vi "SortMessages.vi"() -> ()   [LabVIEW 2020, in "CTI-Peripheral.lvlib"]
uses:
  CTI-Peripheral.lvlib
  Controls/ASCII.ctl
  Controls/ICONS.ctl
  <vilib>/Utility/error.llb/Trim Whitespace One-Sided.vi
panel:
  out "BytesOut 2":u8[](array[numeric]) format="%.0x"
  in  "stop":bool
  out "Shifting ASCII":bool[][](array[boolean])
  out "8x8Text":bool[][](array[boolean])
  in  "Text":string
  out "element":cluster{"BytesOut":u8[]} {"BytesOut" format="%.0x"}
  out "BytesOut":u8[](array[numeric]) format="%.0x"
  in  "ASCII In":bool[][](array[boolean])
  out "ASCII":bool[][](array[boolean])
  out "Boolean array":bool[][](array[boolean])
  in  "Icons":T1
  in  "ASCII":T2
  out "Array":cluster{"BytesOut":u8[]}[](array[cluster])=[{"BytesOut"=[0, 0, 0, 0, 0, 0, 0, 0]}, {"BytesOut"=[24, 0, 24, 24, 60, 60, 24, 0]}, {"BytesOut"=[0, 0, 0, 0, 40, 108, 108, 0]}, {"BytesOut"=[108, 108, 254, 108, 254, 108, 108, 0]}, {"BytesOut"=[16, 60, 64, 56, 4, 120, 16, 0]}, {"BytesOut"=[96, 102, 12, 24, 48, 102, 6, 0]}, {"BytesOut"=[252, 102, 166, 20, 60, 102, 60, 0]}, {"BytesOut"=[0, 0, 0, 12, 24, 24, 24, 0]}, {"BytesOut"=[96, 48, 24, 24, 24, 48, 96, 0]}, {"BytesOut"=[6, 12, 24, 24, 24, 12, 6, 0]}, {"BytesOut"=[0, 108, 56, 254, 56, 108, 0, 0]}, {"BytesOut"=[0, 16, 16, 124, 16, 16, 0, 0]}, {"BytesOut"=[6, 12, 12, 12, 0, 0, 0, 0]}, {"BytesOut"=[0, 0, 0, 60, 0, 0, 0, 0]}, {"BytesOut"=[6, 6, 0, 0, 0, 0, 0, 0]}, {"BytesOut"=[0, 6, 12, 24, 48, 96, 0, 0]}, {"BytesOut"=[28, 34, 34, 34, 34, 34, 34, 28]}, {"BytesOut"=[28, 8, 8, 8, 8, 8, 12, 8]}, {"BytesOut"=[62, 4, 8, 16, 32, 32, 34, 28]}, {"BytesOut"=[28, 34, 32, 32, 24, 32, 34, 28]}, {"BytesOut"=[32, 32, 62, 34, 36, 40, 48, 32]}, {"BytesOut"=[28, 34, 32, 32, 30, 2, 2, 62]}, {"BytesOut"=[28, 34, 34, 34, 30, 2, 34, 28]}, {"BytesOut"=[4, 4, 4, 8, 16, 32, 32, 62]}, {"BytesOut"=[28, 34, 34, 34, 28, 34, 34, 28]}, {"BytesOut"=[28, 34, 32, 60, 34, 34, 34, 28]}, {"BytesOut"=[0, 24, 24, 0, 24, 24, 0, 0]}, {"BytesOut"=[12, 24, 24, 0, 24, 24, 0, 0]}, {"BytesOut"=[96, 48, 24, 12, 24, 48, 96, 0]}, {"BytesOut"=[0, 0, 60, 0, 60, 0, 0, 0]}, {"BytesOut"=[6, 12, 24, 48, 24, 12, 6, 0]}, {"BytesOut"=[24, 0, 24, 56, 96, 102, 60, 0]}, {"BytesOut"=[0, 60, 66, 26, 58, 34, 28, 0]}, {"BytesOut"=[0, 51, 51, 63, 51, 51, 30, 12]}, {"BytesOut"=[0, 63, 102, 102, 62, 102, 102, 63]}, {"BytesOut"=[0, 60, 102, 3, 3, 3, 102, 60]}, {"BytesOut"=[0, 31, 54, 102, 102, 102, 54, 31]}, {"BytesOut"=[0, 127, 70, 22, 30, 22, 70, 127]}, {"BytesOut"=[0, 15, 6, 22, 30, 22, 70, 127]}, {"BytesOut"=[0, 124, 102, 115, 3, 3, 102, 60]}, {"BytesOut"=[0, 51, 51, 51, 63, 51, 51, 51]}, {"BytesOut"=[0, 30, 12, 12, 12, 12, 12, 30]}, {"BytesOut"=[0, 30, 51, 51, 48, 48, 48, 120]}, {"BytesOut"=[0, 103, 102, 54, 30, 54, 102, 103]}, {"BytesOut"=[0, 127, 102, 70, 6, 6, 6, 15]}, {"BytesOut"=[0, 99, 99, 107, 127, 127, 119, 99]}, {"BytesOut"=[0, 99, 99, 115, 123, 111, 103, 99]}, {"BytesOut"=[0, 28, 54, 99, 99, 99, 54, 28]}, {"BytesOut"=[0, 15, 6, 6, 62, 102, 102, 63]}, {"BytesOut"=[0, 56, 30, 59, 51, 51, 51, 30]}, {"BytesOut"=[0, 103, 102, 54, 62, 102, 102, 63]}, {"BytesOut"=[0, 30, 51, 56, 14, 7, 51, 30]}, {"BytesOut"=[0, 30, 12, 12, 12, 12, 45, 63]}, {"BytesOut"=[0, 63, 51, 51, 51, 51, 51, 51]}, {"BytesOut"=[0, 12, 30, 51, 51, 51, 51, 51]}, {"BytesOut"=[0, 99, 119, 127, 107, 99, 99, 99]}, {"BytesOut"=[0, 99, 54, 28, 28, 54, 99, 99]}, {"BytesOut"=[0, 30, 12, 12, 30, 51, 51, 51]}, {"BytesOut"=[0, 127, 102, 76, 24, 49, 99, 127]}, {"BytesOut"=[120, 24, 24, 24, 24, 24, 120, 0]}, {"BytesOut"=[0, 96, 48, 24, 12, 6, 0, 0]}, {"BytesOut"=[30, 24, 24, 24, 24, 24, 30, 0]}, {"BytesOut"=[0, 0, 0, 130, 68, 40, 16, 0]}, {"BytesOut"=[126, 0, 0, 0, 0, 0, 0, 0]}, {"BytesOut"=[0, 0, 0, 0, 96, 48, 48, 0]}, {"BytesOut"=[0, 110, 51, 62, 48, 30, 0, 0]}, {"BytesOut"=[0, 59, 102, 102, 62, 6, 6, 7]}, {"BytesOut"=[0, 30, 51, 3, 51, 30, 0, 0]}, {"BytesOut"=[0, 110, 51, 51, 62, 48, 48, 56]}, {"BytesOut"=[0, 30, 3, 63, 51, 30, 0, 0]}, {"BytesOut"=[0, 15, 6, 6, 15, 6, 54, 28]}, {"BytesOut"=[31, 48, 62, 51, 51, 110, 0, 0]}, {"BytesOut"=[0, 103, 102, 102, 110, 54, 6, 7]}, {"BytesOut"=[0, 30, 12, 12, 12, 14, 0, 12]}, {"BytesOut"=[30, 51, 51, 48, 48, 48, 0, 48]}, {"BytesOut"=[0, 103, 54, 30, 54, 102, 6, 7]}, {"BytesOut"=[0, 30, 12, 12, 12, 12, 12, 14]}, {"BytesOut"=[0, 99, 107, 127, 127, 51, 0, 0]}, {"BytesOut"=[0, 51, 51, 51, 51, 31, 0, 0]}, {"BytesOut"=[0, 30, 51, 51, 51, 30, 0, 0]}, {"BytesOut"=[15, 6, 62, 102, 102, 59, 0, 0]}, {"BytesOut"=[120, 48, 62, 51, 51, 110, 0, 0]}, {"BytesOut"=[0, 15, 6, 102, 110, 59, 0, 0]}, {"BytesOut"=[0, 31, 48, 30, 3, 62, 0, 0]}, {"BytesOut"=[0, 24, 44, 12, 12, 62, 12, 8]}, {"BytesOut"=[0, 110, 51, 51, 51, 51, 0, 0]}, {"BytesOut"=[0, 12, 30, 51, 51, 51, 0, 0]}, {"BytesOut"=[0, 54, 127, 127, 107, 99, 0, 0]}, {"BytesOut"=[0, 99, 54, 28, 54, 99, 0, 0]}, {"BytesOut"=[31, 48, 62, 51, 51, 51, 0, 0]}, {"BytesOut"=[0, 63, 38, 12, 25, 63, 0, 0]}, {"BytesOut"=[112, 24, 24, 12, 24, 24, 112, 0]}, {"BytesOut"=[0, 8, 8, 8, 8, 8, 8, 0]}, {"BytesOut"=[14, 24, 24, 48, 24, 24, 14, 0]}, {"BytesOut"=[0, 0, 0, 54, 92, 0, 0, 0, 0, 0, 0, 0, 0]}] {"BytesOut" format="%.0x"}
  out "unsigned byte array":u8[](array[numeric])
  out "array":string[](array[string])=[" 0x0000000000000000,     // space", "    0x180018183c3c1800,     // !", "    0x00000000286c6c00,     // \"", "    0x6c6cfe6cfe6c6c00,     // #", "    0x103c403804781000,     // $", "    0x60660c1830660600,     // %", "    0xfc66a6143c663c00,     // &", "    0x0000000c18181800,     // '", "    0x6030181818306000,     // (", "    0x060c1818180c0600,     // )", "    0x006c38fe386c0000,     // *", "    0x0010107c10100000,     // +", "    0x060c0c0c00000000,     // ,", "    0x0000003c00000000,     // -", "    0x0606000000000000,     // .", "    0x00060c1830600000,     // /", "    0x1c2222222222221c,     // 0", "    0x1c08080808080c08,     // 1", "    0x3e0408102020221c,     // 2", "    0x1c2220201820221c,     // 3", "    0x20203e2224283020,     // 4", "    0x1c2220201e02023e,     // 5", "    0x1c2222221e02221c,     // 6", "    0x040404081020203e,     // 7", "    0x1c2222221c22221c,     // 8", "    0x1c22203c2222221c,     // 9", "    0x0018180018180000,     // :", "    0x0c18180018180000,     // ;", "    0x6030180c18306000,     // <", "    0x00003c003c000000,     // =", "    0x060c1830180c0600,     // >", "    0x1800183860663c00,     // ?", "    0x003c421a3a221c00,     // @", "    0x0033333f33331e0c,     // A", "    0x003f66663e66663f,     // B", "    0x003c66030303663c,     // C", "    0x001f36666666361f,     // D", "    0x007f46161e16467f,     // E", "    0x000f06161e16467f,     // F", "    0x007c66730303663c,     // G", "    0x003333333f333333,     // H", "    0x001e0c0c0c0c0c1e,     // I", "    0x001e333330303078,     // J", "    0x006766361e366667,     // K", "    0x007f66460606060f,     // L", "    0x0063636b7f7f7763,     // M", "    0x006363737b6f6763,     // N", "    0x001c36636363361c,     // O", "    0x000f06063e66663f,     // P", "    0x00381e3b3333331e,     // Q", "    0x006766363e66663f,     // R", "    0x001e33380e07331e,     // S", "    0x001e0c0c0c0c2d3f,     // T", "    0x003f333333333333,     // U", "    0x000c1e3333333333,     // V", "    0x0063777f6b636363,     // W", "    0x0063361c1c366363,     // X", "    0x001e0c0c1e333333,     // Y", "    0x007f664c1831637f,     // Z", "    0x7818181818187800,     // [", "    0x006030180c060000,     // '\\'", "    0x1e18181818181e00,     // ]", "    0x0000008244281000,     // ^", "    0x7e00000000000000,     // _", "    0x0000000060303000,     // `", "    0x006e333e301e0000,     // a", "    0x003b66663e060607,     // b", "    0x001e3303331e0000,     // c", "    0x006e33333e303038,     // d", "    0x001e033f331e0000,     // e", "    0x000f06060f06361c,     // f", "    0x1f303e33336e0000,     // g", "    0x006766666e360607,     // h", "    0x001e0c0c0c0e000c,     // i", "    0x1e33333030300030,     // j", "    0x0067361e36660607,     // k", "    0x001e0c0c0c0c0c0e,     // l", "    0x00636b7f7f330000,     // m", "    0x00333333331f0000,     // n", "    0x001e3333331e0000,     // o", "    0x0f063e66663b0000,     // p", "    0x78303e33336e0000,     // q", "    0x000f06666e3b0000,     // r", "    0x001f301e033e0000,     // s", "    0x00182c0c0c3e0c08,     // t", "    0x006e333333330000,     // u", "    0x000c1e3333330000,     // v", "    0x00367f7f6b630000,     // w", "    0x0063361c36630000,     // x", "    0x1f303e3333330000,     // y", "    0x003f260c193f0000,     // z", "    0x7018180c18187000,     // {", "    0x0008080808080800,     // |", "    0x0e18183018180e00,     // }", "    0x000000365c000000      // ~"]
  in  "String":string=" 0x0000000000000000,     // space\n    0x180018183c3c1800,     // !\n    0x00000000286c6c00,     // \"\n    0x6c6cfe6cfe6c6c00,     // #\n    0x103c403804781000,     // $\n    0x60660c1830660600,     // %\n    0xfc66a6143c663c00,     // &\n    0x0000000c18181800,     // '\n    0x6030181818306000,     // (\n    0x060c1818180c0600,     // )\n    0x006c38fe386c0000,     // *\n    0x0010107c10100000,     // +\n    0x060c0c0c00000000,     // ,\n    0x0000003c00000000,     // -\n    0x0606000000000000,     // .\n    0x00060c1830600000,     // /\n    0x1c2222222222221c,     // 0\n    0x1c08080808080c08,     // 1\n    0x3e0408102020221c,     // 2\n    0x1c2220201820221c,     // 3\n    0x20203e2224283020,     // 4\n    0x1c2220201e02023e,     // 5\n    0x1c2222221e02221c,     // 6\n    0x040404081020203e,     // 7\n    0x1c2222221c22221c,     // 8\n    0x1c22203c2222221c,     // 9\n    0x0018180018180000,     // :\n    0x0c18180018180000,     // ;\n    0x6030180c18306000,     // <\n    0x00003c003c000000,     // =\n    0x060c1830180c0600,     // >\n    0x1800183860663c00,     // ?\n    0x003c421a3a221c00,     // @\n    0x0033333f33331e0c,     // A\n    0x003f66663e66663f,     // B\n    0x003c66030303663c,     // C\n    0x001f36666666361f,     // D\n    0x007f46161e16467f,     // E\n    0x000f06161e16467f,     // F\n    0x007c66730303663c,     // G\n    0x003333333f333333,     // H\n    0x001e0c0c0c0c0c1e,     // I\n    0x001e333330303078,     // J\n    0x006766361e366667,     // K\n    0x007f66460606060f,     // L\n    0x0063636b7f7f7763,     // M\n    0x006363737b6f6763,     // N\n    0x001c36636363361c,     // O\n    0x000f06063e66663f,     // P\n    0x00381e3b3333331e,     // Q\n    0x006766363e66663f,     // R\n    0x001e33380e07331e,     // S\n    0x001e0c0c0c0c2d3f,     // T\n    0x003f333333333333,     // U\n    0x000c1e3333333333,     // V\n    0x0063777f6b636363,     // W\n    0x0063361c1c366363,     // X\n    0x001e0c0c1e333333,     // Y\n    0x007f664c1831637f,     // Z\n    0x7818181818187800,     // [\n    0x006030180c060000,     // '\\'\n    0x1e18181818181e00,     // ]\n    0x0000008244281000,     // ^\n    0x7e00000000000000,     // _\n    0x0000000060303000,     // `\n    0x006e333e301e0000,     // a\n    0x003b66663e060607,     // b\n    0x001e3303331e0000,     // c\n    0x006e33333e303038,     // d\n    0x001e033f331e0000,     // e\n    0x000f06060f06361c,     // f\n    0x1f303e33336e0000,     // g\n    0x006766666e360607,     // h\n    0x001e0c0c0c0e000c,     // i\n    0x1e33333030300030,     // j\n    0x0067361e36660607,     // k\n    0x001e0c0c0c0c0c0e,     // l\n    0x00636b7f7f330000,     // m\n    0x00333333331f0000,     // n\n    0x001e3333331e0000,     // o\n    0x0f063e66663b0000,     // p\n    0x78303e33336e0000,     // q\n    0x000f06666e3b0000,     // r\n    0x001f301e033e0000,     // s\n    0x00182c0c0c3e0c08,     // t\n    0x006e333333330000,     // u\n    0x000c1e3333330000,     // v\n    0x00367f7f6b630000,     // w\n    0x0063361c36630000,     // x\n    0x1f303e3333330000,     // y\n    0x003f260c193f0000,     // z\n    0x7018180c18187000,     // {\n    0x0008080808080800,     // |\n    0x0e18183018180e00,     // }\n    0x000000365c000000      // ~"
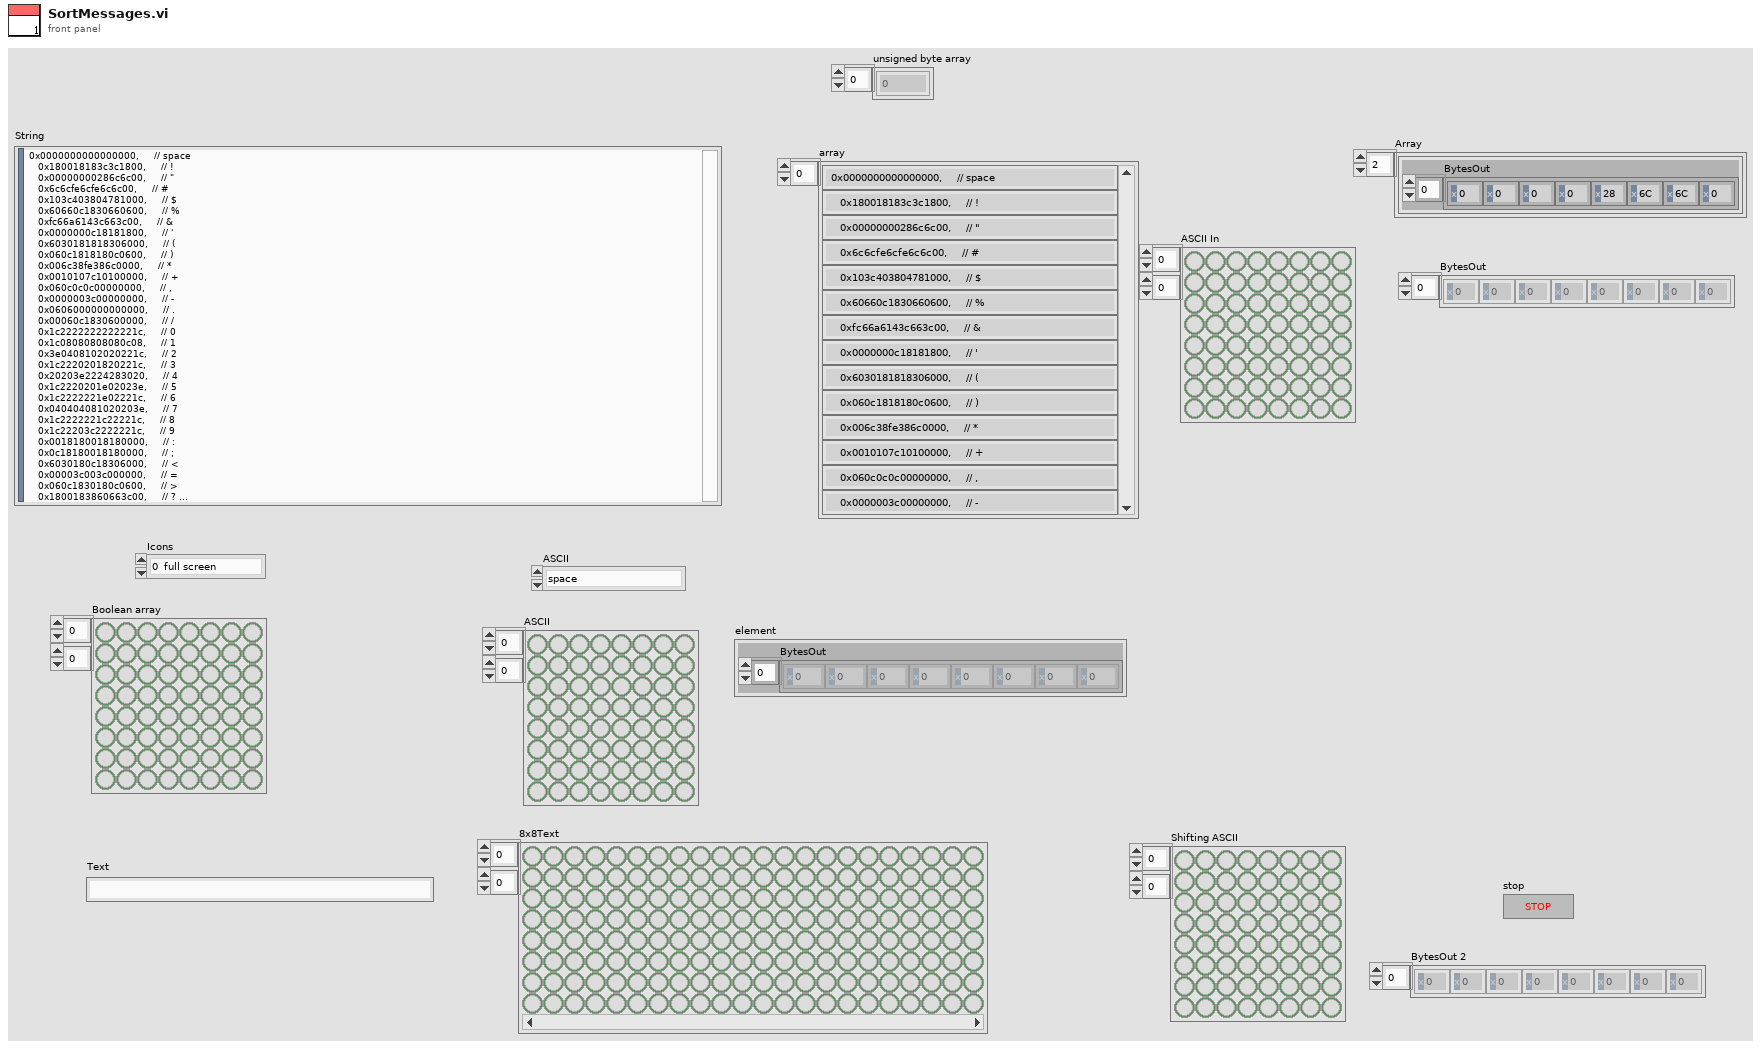
[diagram p1: front panel]
types:
  T1 = typedef "ICONS.ctl" = enum16{"0  full screen", "1  arrow_up", "2  arrow_down", "3  arrow_right", "4  arrow_left", "5  triangle_up", "6  triangle_down", "7  triangle_right", "8  triangel_left", "9  smile_face_1", "10 smile_face_2", "11 hearts", "12 diamonds", "13 clubs", "14 spades", "15 circle1", "16 circle2", "17 circle3", "18 circle4", "19 man", "20 woman", "21 musical_note_1", "22 musical_note_2", "23 snow", "24 up_down", "25 double_!", "26 left_right", "27 house"}
  T2 = typedef "CTI-Peripheral.lvlib/ASCII.ctl" = enum16{"space", "!", "\"", "#", "$", "%", "&", "'", "(", ")", "*", "+", ",", "- ", ".", "/", "0", "1", "2", "3", "4", "5", "6", "7", "8", "9", ":", ";", "<", "=", ">", "?", "@", "A", "B", "C", "D", "E", "F", "G", "H", "I", "J", "K", "L", "M", "N", "O", "P", "Q", "R", "S", "T", "U", "V", "W", "X", "Y", "Z", "[", "'\\'", "]", "^", "_", "`", "a", "b", "c", "d", "e", "f", "g", "h", "i", "j", "k", "l", "m", "n", "o", "p", "q", "r", "s", "t", "u", "v", "w", "x", "y", "z", "{", "|", "}", ""}
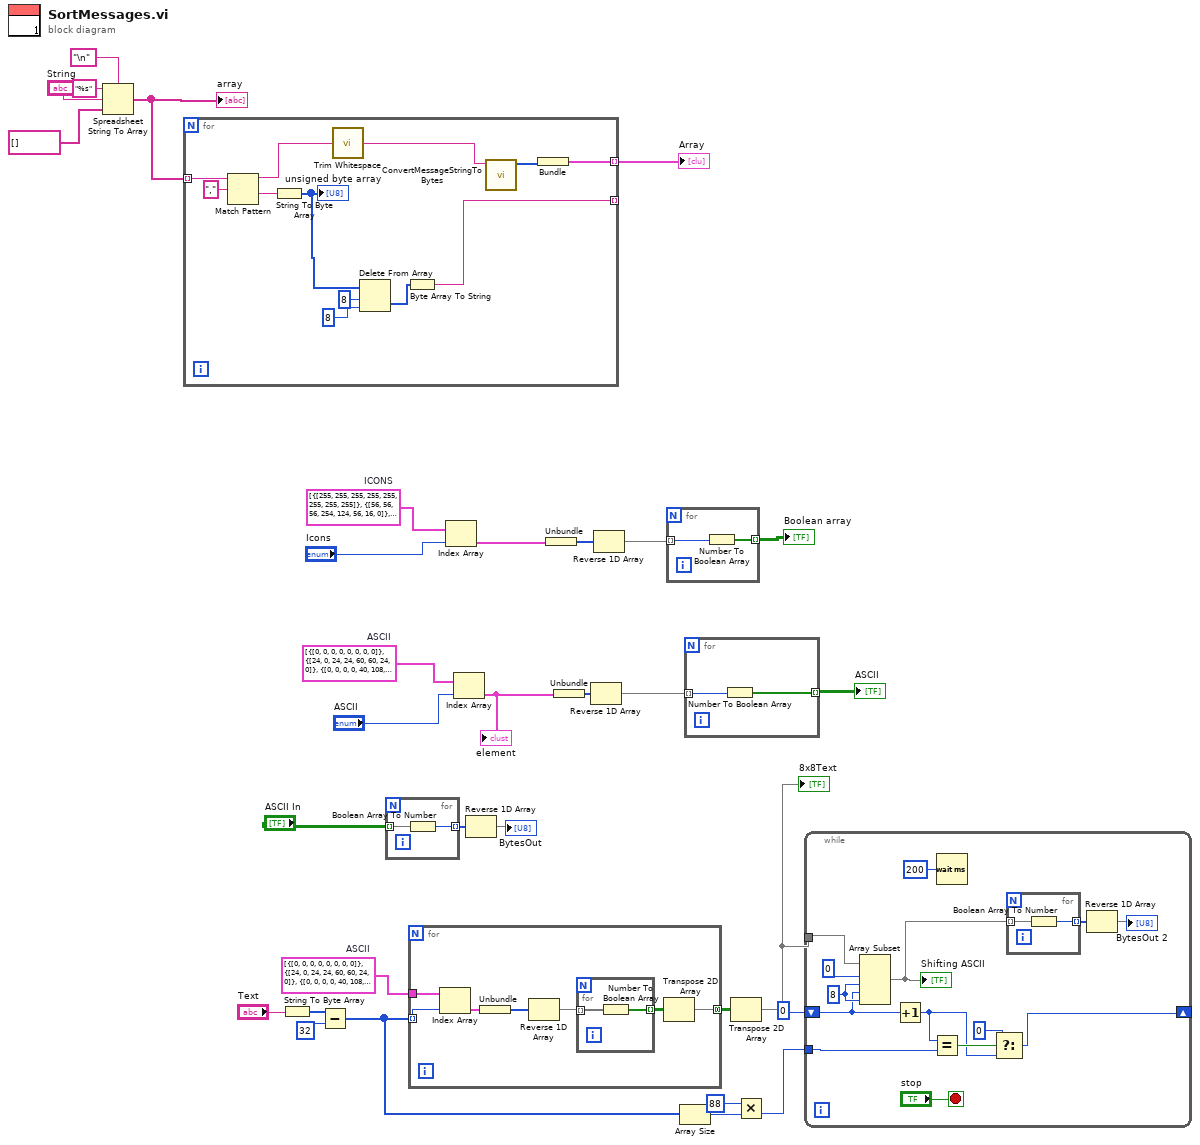
[diagram p0: block diagram]
diagram:
  w8 = cluster{"BytesOut":u8[]}[] [{"BytesOut"=[0, 0, 0, 0, 0, 0, 0, 0]}, {"BytesOut"=[24, 0, 24, 24, 60, 60, 24, 0]}, {"BytesOut"=[0, 0, 0, 0, 40, 108, 108, 0]}, {"BytesOut"=[108, 108, 254, 108, 254, 108, 108, 0]}, {"BytesOut"=[16, 60, 64, 56, 4, 120, 16, 0]}, {"BytesOut"=[96, 102, 12, 24, 48, 102, 6, 0]}, {"BytesOut"=[252, 102, 166, 20, 60, 102, 60, 0]}, {"BytesOut"=[0, 0, 0, 12, 24, 24, 24, 0]}, {"BytesOut"=[96, 48, 24, 24, 24, 48, 96, 0]}, {"BytesOut"=[6, 12, 24, 24, 24, 12, 6, 0]}, {"BytesOut"=[0, 108, 56, 254, 56, 108, 0, 0]}, {"BytesOut"=[0, 16, 16, 124, 16, 16, 0, 0]}, {"BytesOut"=[6, 12, 12, 12, 0, 0, 0, 0]}, {"BytesOut"=[0, 0, 0, 60, 0, 0, 0, 0]}, {"BytesOut"=[6, 6, 0, 0, 0, 0, 0, 0]}, {"BytesOut"=[0, 6, 12, 24, 48, 96, 0, 0]}, {"BytesOut"=[28, 34, 34, 34, 34, 34, 34, 28]}, {"BytesOut"=[28, 8, 8, 8, 8, 8, 12, 8]}, {"BytesOut"=[62, 4, 8, 16, 32, 32, 34, 28]}, {"BytesOut"=[28, 34, 32, 32, 24, 32, 34, 28]}, {"BytesOut"=[32, 32, 62, 34, 36, 40, 48, 32]}, {"BytesOut"=[28, 34, 32, 32, 30, 2, 2, 62]}, {"BytesOut"=[28, 34, 34, 34, 30, 2, 34, 28]}, {"BytesOut"=[4, 4, 4, 8, 16, 32, 32, 62]}, {"BytesOut"=[28, 34, 34, 34, 28, 34, 34, 28]}, {"BytesOut"=[28, 34, 32, 60, 34, 34, 34, 28]}, {"BytesOut"=[0, 24, 24, 0, 24, 24, 0, 0]}, {"BytesOut"=[12, 24, 24, 0, 24, 24, 0, 0]}, {"BytesOut"=[96, 48, 24, 12, 24, 48, 96, 0]}, {"BytesOut"=[0, 0, 60, 0, 60, 0, 0, 0]}, {"BytesOut"=[6, 12, 24, 48, 24, 12, 6, 0]}, {"BytesOut"=[24, 0, 24, 56, 96, 102, 60, 0]}, {"BytesOut"=[0, 60, 66, 26, 58, 34, 28, 0]}, {"BytesOut"=[0, 51, 51, 63, 51, 51, 30, 12]}, {"BytesOut"=[0, 63, 102, 102, 62, 102, 102, 63]}, {"BytesOut"=[0, 60, 102, 3, 3, 3, 102, 60]}, {"BytesOut"=[0, 31, 54, 102, 102, 102, 54, 31]}, {"BytesOut"=[0, 127, 70, 22, 30, 22, 70, 127]}, {"BytesOut"=[0, 15, 6, 22, 30, 22, 70, 127]}, {"BytesOut"=[0, 124, 102, 115, 3, 3, 102, 60]}, {"BytesOut"=[0, 51, 51, 51, 63, 51, 51, 51]}, {"BytesOut"=[0, 30, 12, 12, 12, 12, 12, 30]}, {"BytesOut"=[0, 30, 51, 51, 48, 48, 48, 120]}, {"BytesOut"=[0, 103, 102, 54, 30, 54, 102, 103]}, {"BytesOut"=[0, 127, 102, 70, 6, 6, 6, 15]}, {"BytesOut"=[0, 99, 99, 107, 127, 127, 119, 99]}, {"BytesOut"=[0, 99, 99, 115, 123, 111, 103, 99]}, {"BytesOut"=[0, 28, 54, 99, 99, 99, 54, 28]}, {"BytesOut"=[0, 15, 6, 6, 62, 102, 102, 63]}, {"BytesOut"=[0, 56, 30, 59, 51, 51, 51, 30]}, {"BytesOut"=[0, 103, 102, 54, 62, 102, 102, 63]}, {"BytesOut"=[0, 30, 51, 56, 14, 7, 51, 30]}, {"BytesOut"=[0, 30, 12, 12, 12, 12, 45, 63]}, {"BytesOut"=[0, 63, 51, 51, 51, 51, 51, 51]}, {"BytesOut"=[0, 12, 30, 51, 51, 51, 51, 51]}, {"BytesOut"=[0, 99, 119, 127, 107, 99, 99, 99]}, {"BytesOut"=[0, 99, 54, 28, 28, 54, 99, 99]}, {"BytesOut"=[0, 30, 12, 12, 30, 51, 51, 51]}, {"BytesOut"=[0, 127, 102, 76, 24, 49, 99, 127]}, {"BytesOut"=[120, 24, 24, 24, 24, 24, 120, 0]}, {"BytesOut"=[0, 96, 48, 24, 12, 6, 0, 0]}, {"BytesOut"=[30, 24, 24, 24, 24, 24, 30, 0]}, {"BytesOut"=[0, 0, 0, 130, 68, 40, 16, 0]}, {"BytesOut"=[126, 0, 0, 0, 0, 0, 0, 0]}, {"BytesOut"=[0, 0, 0, 0, 96, 48, 48, 0]}, {"BytesOut"=[0, 110, 51, 62, 48, 30, 0, 0]}, {"BytesOut"=[0, 59, 102, 102, 62, 6, 6, 7]}, {"BytesOut"=[0, 30, 51, 3, 51, 30, 0, 0]}, {"BytesOut"=[0, 110, 51, 51, 62, 48, 48, 56]}, {"BytesOut"=[0, 30, 3, 63, 51, 30, 0, 0]}, {"BytesOut"=[0, 15, 6, 6, 15, 6, 54, 28]}, {"BytesOut"=[31, 48, 62, 51, 51, 110, 0, 0]}, {"BytesOut"=[0, 103, 102, 102, 110, 54, 6, 7]}, {"BytesOut"=[0, 30, 12, 12, 12, 14, 0, 12]}, {"BytesOut"=[30, 51, 51, 48, 48, 48, 0, 48]}, {"BytesOut"=[0, 103, 54, 30, 54, 102, 6, 7]}, {"BytesOut"=[0, 30, 12, 12, 12, 12, 12, 14]}, {"BytesOut"=[0, 99, 107, 127, 127, 51, 0, 0]}, {"BytesOut"=[0, 51, 51, 51, 51, 31, 0, 0]}, {"BytesOut"=[0, 30, 51, 51, 51, 30, 0, 0]}, {"BytesOut"=[15, 6, 62, 102, 102, 59, 0, 0]}, {"BytesOut"=[120, 48, 62, 51, 51, 110, 0, 0]}, {"BytesOut"=[0, 15, 6, 102, 110, 59, 0, 0]}, {"BytesOut"=[0, 31, 48, 30, 3, 62, 0, 0]}, {"BytesOut"=[0, 24, 44, 12, 12, 62, 12, 8]}, {"BytesOut"=[0, 110, 51, 51, 51, 51, 0, 0]}, {"BytesOut"=[0, 12, 30, 51, 51, 51, 0, 0]}, {"BytesOut"=[0, 54, 127, 127, 107, 99, 0, 0]}, {"BytesOut"=[0, 99, 54, 28, 54, 99, 0, 0]}, {"BytesOut"=[31, 48, 62, 51, 51, 51, 0, 0]}, {"BytesOut"=[0, 63, 38, 12, 25, 63, 0, 0]}, {"BytesOut"=[112, 24, 24, 12, 24, 24, 112, 0]}, {"BytesOut"=[0, 8, 8, 8, 8, 8, 8, 0]}, {"BytesOut"=[14, 24, 24, 48, 24, 24, 14, 0]}, {"BytesOut"=[0, 0, 0, 54, 92, 0, 0, 0, 0, 0, 0, 0, 0]}]  # ASCII
  w26 = cluster{"BytesOut":u8[]}[] [{"BytesOut"=[255, 255, 255, 255, 255, 255, 255, 255]}, {"BytesOut"=[56, 56, 56, 254, 124, 56, 16, 0]}, {"BytesOut"=[16, 56, 124, 254, 56, 56, 56, 0]}, {"BytesOut"=[16, 48, 126, 254, 126, 48, 16, 0]}, {"BytesOut"=[16, 24, 252, 254, 252, 24, 16, 0]}, {"BytesOut"=[254, 254, 124, 124, 56, 56, 16, 0]}, {"BytesOut"=[16, 56, 56, 124, 124, 254, 254, 0]}, {"BytesOut"=[6, 30, 126, 254, 126, 30, 6, 0]}, {"BytesOut"=[192, 240, 252, 254, 252, 240, 192, 0]}, {"BytesOut"=[124, 146, 170, 130, 170, 130, 124, 0]}, {"BytesOut"=[0, 60, 66, 0, 0, 102, 0, 0]}, {"BytesOut"=[16, 56, 124, 254, 254, 238, 68, 0]}, {"BytesOut"=[16, 56, 124, 254, 124, 56, 16, 0]}, {"BytesOut"=[56, 16, 84, 254, 84, 56, 16, 0]}, {"BytesOut"=[56, 16, 124, 254, 124, 56, 16, 0]}, {"BytesOut"=[0, 56, 124, 124, 124, 56, 0, 0]}, {"BytesOut"=[255, 199, 131, 131, 131, 199, 255, 255]}, {"BytesOut"=[0, 56, 68, 68, 68, 56, 0, 0]}, {"BytesOut"=[255, 199, 187, 187, 187, 199, 255, 255]}, {"BytesOut"=[12, 18, 18, 156, 160, 192, 240, 0]}, {"BytesOut"=[56, 68, 68, 56, 16, 124, 16, 0]}, {"BytesOut"=[6, 14, 12, 8, 8, 40, 24, 0]}, {"BytesOut"=[6, 110, 236, 200, 136, 152, 240, 0]}, {"BytesOut"=[16, 84, 56, 238, 56, 84, 16, 0]}, {"BytesOut"=[16, 56, 84, 16, 84, 56, 16, 0]}, {"BytesOut"=[102, 102, 0, 102, 102, 102, 102, 0]}, {"BytesOut"=[0, 40, 68, 254, 68, 40, 0, 0]}, {"BytesOut"=[254, 130, 130, 198, 108, 56, 16, 0]}, {"BytesOut"=[0, 36, 0, 231, 165, 189, 231, 0, 0, 0, 0, 0, 2, 8, 0, 10, 0]}]  # ICONS
  w19 = cluster{"BytesOut":u8[]}[] [{"BytesOut"=[0, 0, 0, 0, 0, 0, 0, 0]}, {"BytesOut"=[24, 0, 24, 24, 60, 60, 24, 0]}, {"BytesOut"=[0, 0, 0, 0, 40, 108, 108, 0]}, {"BytesOut"=[108, 108, 254, 108, 254, 108, 108, 0]}, {"BytesOut"=[16, 60, 64, 56, 4, 120, 16, 0]}, {"BytesOut"=[96, 102, 12, 24, 48, 102, 6, 0]}, {"BytesOut"=[252, 102, 166, 20, 60, 102, 60, 0]}, {"BytesOut"=[0, 0, 0, 12, 24, 24, 24, 0]}, {"BytesOut"=[96, 48, 24, 24, 24, 48, 96, 0]}, {"BytesOut"=[6, 12, 24, 24, 24, 12, 6, 0]}, {"BytesOut"=[0, 108, 56, 254, 56, 108, 0, 0]}, {"BytesOut"=[0, 16, 16, 124, 16, 16, 0, 0]}, {"BytesOut"=[6, 12, 12, 12, 0, 0, 0, 0]}, {"BytesOut"=[0, 0, 0, 60, 0, 0, 0, 0]}, {"BytesOut"=[6, 6, 0, 0, 0, 0, 0, 0]}, {"BytesOut"=[0, 6, 12, 24, 48, 96, 0, 0]}, {"BytesOut"=[28, 34, 34, 34, 34, 34, 34, 28]}, {"BytesOut"=[28, 8, 8, 8, 8, 8, 12, 8]}, {"BytesOut"=[62, 4, 8, 16, 32, 32, 34, 28]}, {"BytesOut"=[28, 34, 32, 32, 24, 32, 34, 28]}, {"BytesOut"=[32, 32, 62, 34, 36, 40, 48, 32]}, {"BytesOut"=[28, 34, 32, 32, 30, 2, 2, 62]}, {"BytesOut"=[28, 34, 34, 34, 30, 2, 34, 28]}, {"BytesOut"=[4, 4, 4, 8, 16, 32, 32, 62]}, {"BytesOut"=[28, 34, 34, 34, 28, 34, 34, 28]}, {"BytesOut"=[28, 34, 32, 60, 34, 34, 34, 28]}, {"BytesOut"=[0, 24, 24, 0, 24, 24, 0, 0]}, {"BytesOut"=[12, 24, 24, 0, 24, 24, 0, 0]}, {"BytesOut"=[96, 48, 24, 12, 24, 48, 96, 0]}, {"BytesOut"=[0, 0, 60, 0, 60, 0, 0, 0]}, {"BytesOut"=[6, 12, 24, 48, 24, 12, 6, 0]}, {"BytesOut"=[24, 0, 24, 56, 96, 102, 60, 0]}, {"BytesOut"=[0, 60, 66, 26, 58, 34, 28, 0]}, {"BytesOut"=[0, 51, 51, 63, 51, 51, 30, 12]}, {"BytesOut"=[0, 63, 102, 102, 62, 102, 102, 63]}, {"BytesOut"=[0, 60, 102, 3, 3, 3, 102, 60]}, {"BytesOut"=[0, 31, 54, 102, 102, 102, 54, 31]}, {"BytesOut"=[0, 127, 70, 22, 30, 22, 70, 127]}, {"BytesOut"=[0, 15, 6, 22, 30, 22, 70, 127]}, {"BytesOut"=[0, 124, 102, 115, 3, 3, 102, 60]}, {"BytesOut"=[0, 51, 51, 51, 63, 51, 51, 51]}, {"BytesOut"=[0, 30, 12, 12, 12, 12, 12, 30]}, {"BytesOut"=[0, 30, 51, 51, 48, 48, 48, 120]}, {"BytesOut"=[0, 103, 102, 54, 30, 54, 102, 103]}, {"BytesOut"=[0, 127, 102, 70, 6, 6, 6, 15]}, {"BytesOut"=[0, 99, 99, 107, 127, 127, 119, 99]}, {"BytesOut"=[0, 99, 99, 115, 123, 111, 103, 99]}, {"BytesOut"=[0, 28, 54, 99, 99, 99, 54, 28]}, {"BytesOut"=[0, 15, 6, 6, 62, 102, 102, 63]}, {"BytesOut"=[0, 56, 30, 59, 51, 51, 51, 30]}, {"BytesOut"=[0, 103, 102, 54, 62, 102, 102, 63]}, {"BytesOut"=[0, 30, 51, 56, 14, 7, 51, 30]}, {"BytesOut"=[0, 30, 12, 12, 12, 12, 45, 63]}, {"BytesOut"=[0, 63, 51, 51, 51, 51, 51, 51]}, {"BytesOut"=[0, 12, 30, 51, 51, 51, 51, 51]}, {"BytesOut"=[0, 99, 119, 127, 107, 99, 99, 99]}, {"BytesOut"=[0, 99, 54, 28, 28, 54, 99, 99]}, {"BytesOut"=[0, 30, 12, 12, 30, 51, 51, 51]}, {"BytesOut"=[0, 127, 102, 76, 24, 49, 99, 127]}, {"BytesOut"=[120, 24, 24, 24, 24, 24, 120, 0]}, {"BytesOut"=[0, 96, 48, 24, 12, 6, 0, 0]}, {"BytesOut"=[30, 24, 24, 24, 24, 24, 30, 0]}, {"BytesOut"=[0, 0, 0, 130, 68, 40, 16, 0]}, {"BytesOut"=[126, 0, 0, 0, 0, 0, 0, 0]}, {"BytesOut"=[0, 0, 0, 0, 96, 48, 48, 0]}, {"BytesOut"=[0, 110, 51, 62, 48, 30, 0, 0]}, {"BytesOut"=[0, 59, 102, 102, 62, 6, 6, 7]}, {"BytesOut"=[0, 30, 51, 3, 51, 30, 0, 0]}, {"BytesOut"=[0, 110, 51, 51, 62, 48, 48, 56]}, {"BytesOut"=[0, 30, 3, 63, 51, 30, 0, 0]}, {"BytesOut"=[0, 15, 6, 6, 15, 6, 54, 28]}, {"BytesOut"=[31, 48, 62, 51, 51, 110, 0, 0]}, {"BytesOut"=[0, 103, 102, 102, 110, 54, 6, 7]}, {"BytesOut"=[0, 30, 12, 12, 12, 14, 0, 12]}, {"BytesOut"=[30, 51, 51, 48, 48, 48, 0, 48]}, {"BytesOut"=[0, 103, 54, 30, 54, 102, 6, 7]}, {"BytesOut"=[0, 30, 12, 12, 12, 12, 12, 14]}, {"BytesOut"=[0, 99, 107, 127, 127, 51, 0, 0]}, {"BytesOut"=[0, 51, 51, 51, 51, 31, 0, 0]}, {"BytesOut"=[0, 30, 51, 51, 51, 30, 0, 0]}, {"BytesOut"=[15, 6, 62, 102, 102, 59, 0, 0]}, {"BytesOut"=[120, 48, 62, 51, 51, 110, 0, 0]}, {"BytesOut"=[0, 15, 6, 102, 110, 59, 0, 0]}, {"BytesOut"=[0, 31, 48, 30, 3, 62, 0, 0]}, {"BytesOut"=[0, 24, 44, 12, 12, 62, 12, 8]}, {"BytesOut"=[0, 110, 51, 51, 51, 51, 0, 0]}, {"BytesOut"=[0, 12, 30, 51, 51, 51, 0, 0]}, {"BytesOut"=[0, 54, 127, 127, 107, 99, 0, 0]}, {"BytesOut"=[0, 99, 54, 28, 54, 99, 0, 0]}, {"BytesOut"=[31, 48, 62, 51, 51, 51, 0, 0]}, {"BytesOut"=[0, 63, 38, 12, 25, 63, 0, 0]}, {"BytesOut"=[112, 24, 24, 12, 24, 24, 112, 0]}, {"BytesOut"=[0, 8, 8, 8, 8, 8, 8, 0]}, {"BytesOut"=[14, 24, 24, 48, 24, 24, 14, 0]}, {"BytesOut"=[0, 0, 0, 54, 92, 0, 0, 0, 0, 0, 0, 0, 0]}]  # ASCII
  n1 = Spreadsheet String To Array(delimiter (Tab)="\n", format string="%s", spreadsheet string="String", array type (2D Dbl)=string[] []) -> (array=w28:string[])
  "array" <- w28
  n2 = for {
    tunnel: w28 -> [w44] mode=indexing
    tunnel: [w38] -> _ mode=indexing
    tunnel: [w33] -> w27 mode=indexing
    n3 = Match Pattern(string=w44, regular expression=",") -> (before substring=w42:string, after substring=w41:string)  [unwired: 1 in, 2 out]
    n4 = String To Byte Array(string=w41) -> (unsigned byte array=w40:u8[])
    "unsigned byte array" <- w40
    n5 = call <vilib>:"Trim Whitespace.vi"("string"=w42) -> ("trimmed string"=w35:string)  [unwired: 1 in]
    n6 = Delete From Array(array=w40, length=8, index=8) -> (deleted portion=w36:u8[])  [unwired: 1 out]
    n7 = Byte Array To String(unsigned byte array=w36) -> (string=w38:string)
    n8 = call "ConvertMessageStringToBytes.vi"("8x8MessageString"=w35) -> ("BytesOut"=w34:u8[])  [unwired: 10 in]
    n9 = Bundle("BytesOut"=w34) -> (w33:cluster{"BytesOut":u8[]})  [unwired: 1 in]
  }
  "Array" <- w27
  n10 = String To Byte Array(string="Text") -> (unsigned byte array=w10:u8[])
  n11 = Subtract(x=w10, y=32) -> (x-y=w7:i32[])
  n12 = for {
    tunnel: "ASCII In" -> [w46] mode=indexing
    tunnel: [w45] -> w14 mode=indexing
    n13 = Boolean Array To Number(Boolean array=w46) -> (number=w45:u32)
  }
  n14 = for {
    tunnel: w7 -> [w53] mode=indexing
    tunnel: w8 -> [w52]
    tunnel: [w48] -> w4 mode=concatenating
    n15 = Index Array(array=w52, index=w53) -> (element=w51:cluster{"BytesOut":u8[]})
    n16 = Unbundle(w51) -> ("BytesOut"=w49:u8[])
    n17 = Reverse 1D Array(array=w49) -> (reversed array=w47:u8[])
    n18 = for {
      tunnel: w47 -> [w55] mode=indexing
      tunnel: [w54] -> w50 mode=indexing
      n19 = Number To Boolean Array(number=w55) -> (Boolean array=w54:bool[])
    }
    n20 = Transpose 2D Array(2D array=w50) -> (transposed array=w48:bool[][])
  }
  n21 = Index Array(array=w26, index="Icons") -> (element=w24:cluster{"BytesOut":u8[]})
  n22 = Index Array(array=w19, index="ASCII") -> (element=w20:cluster{"BytesOut":u8[]})
  "element" <- w20
  n23 = Reverse 1D Array(array=w14) -> (reversed array=→"BytesOut":u32[])
  n24 = Unbundle(w24) -> ("BytesOut"=w23:u8[])
  n25 = Unbundle(w20) -> ("BytesOut"=w21:u8[])
  n26 = Reverse 1D Array(array=w21) -> (reversed array=w15:u8[])
  n27 = Reverse 1D Array(array=w23) -> (reversed array=w17:u8[])
  n28 = for {
    tunnel: w17 -> [w57] mode=indexing
    tunnel: [w56] -> w16 mode=indexing
    n29 = Number To Boolean Array(number=w57) -> (Boolean array=w56:bool[])
  }
  "Boolean array" <- w16
  n30 = Array Size(array=w7) -> (size(s)=w6:i32)
  n31 = for {
    tunnel: w15 -> [w59] mode=indexing
    tunnel: [w58] -> w22 mode=indexing
    n32 = Number To Boolean Array(number=w59) -> (Boolean array=w58:bool[])
  }
  "ASCII" <- w22
  n33 = Transpose 2D Array(2D array=w4) -> (transposed array=w3:bool[][])
  "8x8Text" <- w3
  n34 = Multiply(x=88, y=w6) -> (x*y=w2:i32)
  n35 = while {
    tunnel: w3 -> [w73]
    tunnel: w2 -> [w70]
    shift-right: [w66] -> _
    shift-left: 0 ("index") -> [w63]
    stop <- "stop" stop-if-true
    w65 = 8 ("length")
    n36 = Array Subset(array=w73, index (row)=0 ("index"), length (row)=w65, index (col)=w63, length (col)=w65) -> (w60:bool[][])
    "Shifting ASCII" <- w60
    n37 = Increment(x=w63) -> (x+1=w68:i32)
    n38 = Equal?(x=w68, y=w70) -> (x = y?=w69:bool)
    n39 = Wait (ms)(milliseconds to wait=u32 200) -> ()  [unwired: 1 out]
    n40 = Select(t=0 ("index"), s=w69, f=w68) -> (s? t:f=w66:i32)
    n41 = for {
      tunnel: w60 -> [w75] mode=indexing
      tunnel: [w74] -> w61 mode=indexing
      n42 = Boolean Array To Number(Boolean array=w75) -> (number=w74:u32)
    }
    n43 = Reverse 1D Array(array=w61) -> (reversed array=→"BytesOut 2":u32[])
  }
